vi "movestuff.vi"() -> ()   [LabVIEW 2017]
doc: "\"Discrete LED demo.vi\" -- Demonstrate a discrete LED connected to a digital output.\n\nInstructions:\n\n-- Click the 'enable blinker' button to toggle between blinking mode\nand static mode.\n-- In static mode, click the 'digital level' button to set the state of the\ndigital output.\n-- The 'digital output state' LED indicator shows the state of the\ndigital output (on = high, off = low)."
uses:
  <vilib>/myRIO/Instrument Drivers/Onboard IO/PWM/typedefs/PWM Reference.ctl
  <vilib>/myRIO/Common/Instrument Driver Framework/Utilities/typedefs/myRIO Generic Hardware Reference.ctl
  <vilib>/myRIO/Common/Instrument Driver Framework/Utilities/typedefs/Hardware Version Enum.ctl
  <vilib>/myRIO/Common/Instrument Driver Framework/Utilities/typedefs/myRIO v1.0 Reference.ctl
  <vilib>/myRIO/Common/Instrument Driver Framework/Utilities/typedefs/Generic FPGA Reference.ctl
  <vilib>/myRIO/Common/Instrument Driver Framework/myRIO v1.0/PWM/typedefs/PWM Channels Enum.ctl
  <vilib>/myRIO/Instrument Drivers/Onboard IO/PWM/typedefs/PWM Configuration.ctl
  <vilib>/userdefined/High Color/nirio_resource_hc.ctl
  <vilib>/myRIO/Instrument Drivers/Onboard IO/DIO/typedefs/DIO Reference.ctl
  <vilib>/myRIO/Common/Instrument Driver Framework/myRIO v1.0/DIO/typedefs/DIO Channels List.ctl
  <vilib>/myRIO/Common/Instrument Driver Framework/myRIO v1.0/DIO/typedefs/DIO Channels Enum.ctl
  <vilib>/myRIO/Common/Instrument Driver Framework/Utilities/vis/Is FPGA Ref Available.vi
  <vilib>/myRIO/Common/Instrument Driver Framework/myRIO v1.0/PWM/vis/myRIO v1.1 Open PWM.vi
  <vilib>/myRIO/Instrument Drivers/Onboard IO/PWM/vis/Set Duty Cycle and Frequency.vi
  <vilib>/myRIO/Common/Instrument Driver Framework/myRIO v1.0/DIO/vis/myRIO v1.1 Open DIO.vi
  <vilib>/myRIO/Instrument Drivers/Onboard IO/DIO/vis/Write.vi
  <vilib>/myRIO/Common/Instrument Driver Framework/Utilities/vis/Validate Channels.vi
  <vilib>/myRIO/Common/Instrument Driver Framework/myRIO v1.0/PWM/vis/myRIO v1.0 Reserve PWM.vi
  <vilib>/myRIO/Common/Instrument Driver Framework/myRIO v1.0/DIO/vis/myRIO v1.0 Reserve DIO.vi
  <vilib>/myRIO/Common/Instrument Driver Framework/myRIO v1.0/UART/vis/myRIO v1.0 Close UART.vi
  <vilib>/myRIO/Common/Instrument Driver Framework/myRIO v1.0/PWM/vis/myRIO v1.0 Build MUX Configuration PWM.vi
  <vilib>/myRIO/Common/Instrument Driver Framework/myRIO v1.0/Resource Manager/vis/myRIO v1.0 Reserve Channel List.vi
  <vilib>/myRIO/Common/Instrument Driver Framework/myRIO v1.0/DIO/vis/myRIO v1.0 Build MUX Configuration DIO.vi
  <vilib>/myRIO/Common/Instrument Driver Framework/myRIO v1.0/Resource Manager/vis/myRIO v1.0 Create Configuration List.vi
  <vilib>/myRIO/Common/Instrument Driver Framework/myRIO v1.0/Resource Manager/vis/myRIO v1.0 Reserve Channel.vi
  <vilib>/myRIO/Common/Instrument Driver Framework/myRIO v1.0/Resource Manager/vis/myRIO v1.0 Unreserve Channel.vi
  <vilib>/myRIO/Common/Instrument Driver Framework/myRIO v1.0/Resource Manager/vis/myRIO v1.0 Build Mutex Name.vi
  <vilib>/Utility/VariantDataType/GetNumericInfo.vi
  <vilib>/Utility/error.llb/Error Cluster From Error Code.vi
  <vilib>/myRIO/Common/Instrument Driver Framework/myRIO v1.0/myRIO v1.1 Open.vi
  <vilib>/myRIO/Common/Instrument Driver Framework/Utilities/vis/IO Manager.vi
  <vilib>/myRIO/Common/Instrument Driver Framework/Utilities/vis/Configuration Manager.vi
  <vilib>/myRIO/Common/Instrument Driver Framework/myRIO v1.0/Resource Manager/vis/myRIO v1.0 Configure IO.vi
  <vilib>/myRIO/Common/Instrument Driver Framework/myRIO v1.0/myRIO v1.0 Close.vi
  <vilib>/myRIO/Common/Instrument Driver Framework/myRIO v1.0/PWM/vis/myRIO v1.0 Write PWM.vi
  <vilib>/myRIO/Common/Instrument Driver Framework/myRIO v1.0/DIO/vis/myRIO v1.0 Write DIO.vi
  <vilib>/myRIO/Common/Instrument Driver Framework/Utilities/vis/FPGA Ref Manager.vi
  <vilib>/myRIO/Common/Instrument Driver Framework/myRIO v1.0/myRIO v1.0 Reset FPGA.vi
  <vilib>/myRIO/Common/Instrument Driver Framework/myRIO v1.0/IRQ/vis/myRIO v1.0 IRQ Info FGV.vi
  <vilib>/myRIO/Common/Instrument Driver Framework/myRIO v1.0/IRQ/vis/myRIO v1.0 Timer IRQ Info FGV.vi
  <vilib>/myRIO/Common/Instrument Driver Framework/myRIO v1.0/IRQ/vis/myRIO v1.0 ISR Agent.vi
  <vilib>/myRIO/Express VI/Onboard IO/PWM/PWM Express VI.xnode
  <vilib>/myRIO/Instrument Drivers/Onboard IO/PWM/vis/myRIO PWM Open.xnode
  <vilib>/myRIO/Express VI/Onboard Devices/LED/LED Express VI.xnode
  <vilib>/myRIO/Instrument Drivers/Onboard IO/DIO/vis/myRIO DIO Open.xnode
  <vilib>/myRIO/Express VI/Onboard IO/DO/DO Express VI.xnode
  <vilib>/myRIO/Instrument Drivers/Utilities/Utilities.lvlib
  <vilib>/myRIO/Instrument Drivers/Onboard IO/PWM/PWM.lvlib
  <vilib>/myRIO/Instrument Drivers/Onboard IO/DIO/DIO.lvlib
panel:
  in  "PWM 2":dbl(slide)=0.5 scale=0.0..1.0
  in  "PWM 1":dbl(slide)=0.5 scale=0.0..1.0
  in  "Stop Button":bool
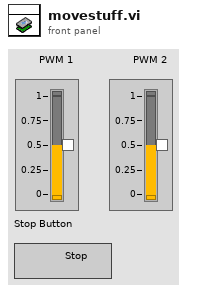
[diagram p1: front panel]
types:
  T1 = typedef "DIO.lvlib/DIO Reference.ctl" = cluster{"myRIO Reference":T2, "DIO Channels List":T6}
  T2 = typedef "myRIO Generic Hardware Reference.ctl" = cluster{"myRIO Model":T3, "myRIO Hardware Reference":T4}
  T3 = typedef "Hardware Version Enum.ctl" = enum16{"Unknown", "myRIO-1900", "myRIO-1950", "roboRIO", "NI ELVIS RIO CM"}
  T4 = typedef "myRIO v1.0 Reference.ctl" = cluster{"Generic FPGA Reference":T5, "Allow multiple opens":bool}
  T5 = typedef "Generic FPGA Reference.ctl" = refnum<k20>
  T6 = typedef "DIO Channels List.ctl" = T7[]
  T7 = typedef "DIO Channels Enum.ctl" = enum16{"Not Connected", "C/DIO0", "C/DIO1", "C/DIO2", "C/DIO3", "C/DIO4", "C/DIO5", "C/DIO6", "C/DIO7", "A/DIO0", "A/DIO1", "A/DIO2", "A/DIO3", "A/DIO4", "A/DIO5", "A/DIO6", "A/DIO7", "A/DIO8", "A/DIO9", "A/DIO10", "A/DIO11", "A/DIO12", "A/DIO13", "A/DIO14", "A/DIO15", "B/DIO0", "B/DIO1", "B/DIO2", "B/DIO3", "B/DIO4", "B/DIO5", "B/DIO6", "B/DIO7", "B/DIO8", "B/DIO9", "B/DIO10", "B/DIO11", "B/DIO12", "B/DIO13", "B/DIO14", "B/DIO15", "LED0", "LED1", "LED2", "LED3", "Button0", "DIO/DIO0", "DIO/DIO1", "DIO/DIO2", "DIO/DIO3", "DIO/DIO4", "DIO/DIO5", "DIO/DIO6", "DIO/DIO7", "DIO/DIO8", "DIO/DIO9", "SPI/CS0", "SPI/CS1", "SPI/CS2", "SPI/CS3", "LED RADIO (Green)", "LED RADIO (Red)", "LED COMM (Green)", "LED COMM (Red)", "LED MODE (Green)", "LED MODE (Red)"}
  T8 = typedef "nirio_resource_hc.ctl" = tag
  T9 = typedef "PWM.lvlib/PWM Reference.ctl" = cluster{"myRIO Reference":T2, "PWM Channels Enum":T10, "PWM Configuration":T11}
  T10 = typedef "PWM Channels Enum.ctl" = enum16{"Not Connected", "C/PWM0", "C/PWM1", "A/PWM0", "A/PWM1", "A/PWM2", "B/PWM0", "B/PWM1", "B/PWM2", "PWM/PWM0", "PWM/PWM1", "PWM/PWM2", "PWM/PWM3", "PWM/PWM4", "PWM/PWM5", "PWM/PWM6", "PWM/PWM7", "PWM/PWM8", "PWM/PWM9"}
  T11 = typedef "PWM.lvlib/PWM Configuration.ctl" = cluster{"Frequency":dbl, "Duty Cycle":dbl}
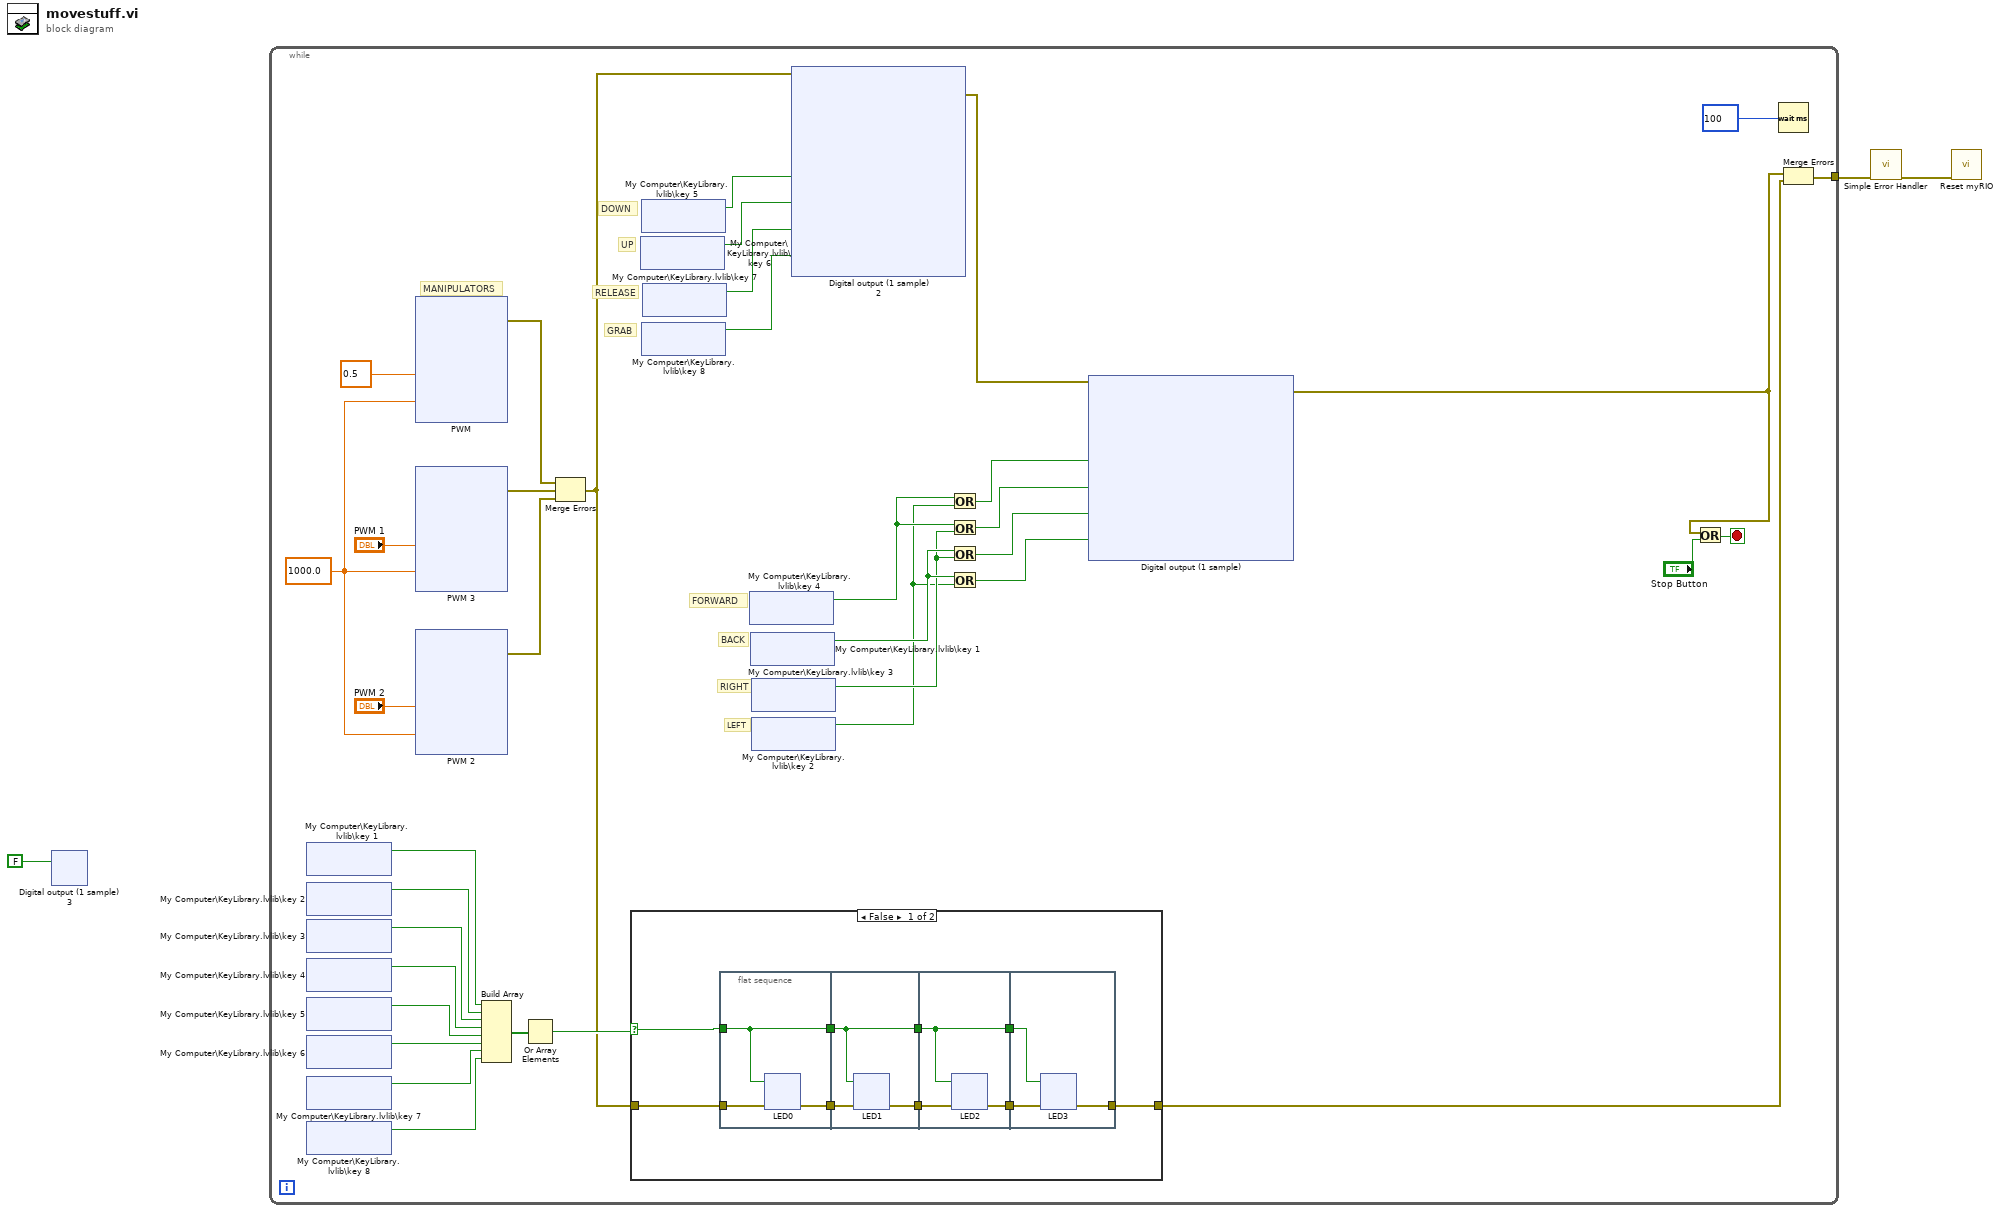
[diagram p0: block diagram]
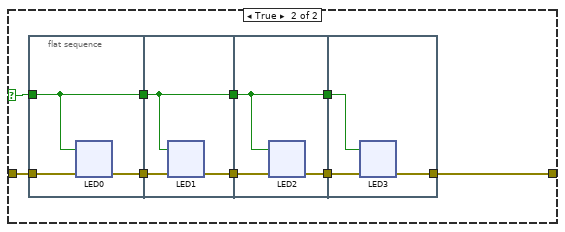
[diagram p2: hidden frame]
diagram:
  n1 = xnode "Digital output (1 sample) 3"("LED_pos (A/DIO2 (Pin 15))"=FALSE) -> ()  [unwired: 1 in, 1 out]
  n2 = while {
    tunnel: [w15] -> w2
    stop <- w39 stop-if-true
    w30 = 1000.0 ("Frequency [Hz]")
    # "RELEASE"
    # "GRAB"
    # "DOWN"
    # "UP"
    # "LEFT"
    # "RIGHT"
    # "BACK"
    # "FORWARD"
    # "MANIPULATORS"
    n3 = shared-variable "My Computer\\KeyLibrary.lvlib\\key 1"() -> (w25:bool)  [unwired: 1 in, 1 out]
    n4 = shared-variable "My Computer\\KeyLibrary.lvlib\\key 2"() -> (w24:bool)  [unwired: 1 in, 1 out]
    n5 = shared-variable "My Computer\\KeyLibrary.lvlib\\key 3"() -> (w23:bool)  [unwired: 1 in, 1 out]
    n6 = shared-variable "My Computer\\KeyLibrary.lvlib\\key 4"() -> (w22:bool)  [unwired: 1 in, 1 out]
    n7 = shared-variable "My Computer\\KeyLibrary.lvlib\\key 5"() -> (w21:bool)  [unwired: 1 in, 1 out]
    n8 = shared-variable "My Computer\\KeyLibrary.lvlib\\key 6"() -> (w20:bool)  [unwired: 1 in, 1 out]
    n9 = shared-variable "My Computer\\KeyLibrary.lvlib\\key 7"() -> (w19:bool)  [unwired: 1 in, 1 out]
    n10 = shared-variable "My Computer\\KeyLibrary.lvlib\\key 8"() -> (w18:bool)  [unwired: 1 in, 1 out]
    n11 = xnode "PWM"("Duty Cycle"=0.5, "Frequency [Hz]"=w30) -> ("error out"=w35:errorcluster)  [unwired: 1 in]
    n12 = xnode "PWM 3"("Duty Cycle"="PWM 1", "Frequency [Hz]"=w30) -> ("error out"=w38:errorcluster)  [unwired: 1 in]
    n13 = xnode "PWM 2"("Duty Cycle"="PWM 2", "Frequency [Hz]"=w30) -> ("error out"=w37:errorcluster)  [unwired: 1 in]
    n14 = Build Array(w25, w24, w23, w22, w21, w20, w19, w18) -> (w17:bool[])
    n15 = Or Array Elements(Boolean array=w17) -> (logical OR=w16:bool)
    n16 = Merge Errors(w35, w38, w37) -> (w13:errorcluster)
    n17 = case shown="False" w16 {
      selector: w16 -> [w41 w210]
      tunnel: [w42 w202] -> w14
      tunnel: w13 -> [w43 w203]
      frame False {
        n18 = flat-sequence {
          tunnel: w41 -> [w50]
          tunnel: [w50] -> w49
          tunnel: [w52] -> w48
          tunnel: w43 -> [w51]
          tunnel: [w90] -> w47
          tunnel: w49 -> [w90]
          tunnel: w48 -> [w89]
          tunnel: [w88] -> w46
          tunnel: [w128] -> w45
          tunnel: w47 -> [w128]
          tunnel: w46 -> [w127]
          tunnel: [w126] -> w44
          tunnel: w45 -> [w166]
          tunnel: w44 -> [w165]
          tunnel: [w164] -> w42
          frame #0 {
            n19 = xnode "LED0"("error in (no error)"=w51, "LED0"=w50) -> ("error out"=w52:errorcluster)
          }
          frame #1 {
            n20 = xnode "LED1"("error in (no error)"=w89, "LED1"=w90) -> ("error out"=w88:errorcluster)
          }
          frame #2 {
            n21 = xnode "LED2"("error in (no error)"=w127, "LED2"=w128) -> ("error out"=w126:errorcluster)
          }
          frame #3 {
            n22 = xnode "LED3"("error in (no error)"=w165, "LED3"=w166) -> ("error out"=w164:errorcluster)
          }
        }
      }
      frame True {
        n23 = flat-sequence {
          tunnel: w210 -> [w213]
          tunnel: [w213] -> w207
          tunnel: [w212] -> w206
          tunnel: w203 -> [w211]
          tunnel: [w251] -> w208
          tunnel: w207 -> [w251]
          tunnel: w206 -> [w250]
          tunnel: [w249] -> w205
          tunnel: [w289] -> w209
          tunnel: w208 -> [w289]
          tunnel: w205 -> [w288]
          tunnel: [w287] -> w204
          tunnel: w209 -> [w327]
          tunnel: w204 -> [w326]
          tunnel: [w325] -> w202
          frame #0 {
            n24 = xnode "LED0"("error in (no error)"=w211, "LED0"=w213) -> ("error out"=w212:errorcluster)
          }
          frame #1 {
            n25 = xnode "LED1"("error in (no error)"=w250, "LED1"=w251) -> ("error out"=w249:errorcluster)
          }
          frame #2 {
            n26 = xnode "LED2"("error in (no error)"=w288, "LED2"=w289) -> ("error out"=w287:errorcluster)
          }
          frame #3 {
            n27 = xnode "LED3"("error in (no error)"=w326, "LED3"=w327) -> ("error out"=w325:errorcluster)
          }
        }
      }
    }
    n28 = shared-variable "My Computer\\KeyLibrary.lvlib\\key 6"() -> (w6:bool)  [unwired: 1 in, 1 out]
    n29 = shared-variable "My Computer\\KeyLibrary.lvlib\\key 5"() -> (w7:bool)  [unwired: 1 in, 1 out]
    n30 = shared-variable "My Computer\\KeyLibrary.lvlib\\key 8"() -> (w4:bool)  [unwired: 1 in, 1 out]
    n31 = shared-variable "My Computer\\KeyLibrary.lvlib\\key 7"() -> (w5:bool)  [unwired: 1 in, 1 out]
    n32 = shared-variable "My Computer\\KeyLibrary.lvlib\\key 4"() -> (w29:bool)  [unwired: 1 in, 1 out]
    n33 = shared-variable "My Computer\\KeyLibrary.lvlib\\key 1"() -> (w28:bool)  [unwired: 1 in, 1 out]
    n34 = shared-variable "My Computer\\KeyLibrary.lvlib\\key 3"() -> (w9:bool)  [unwired: 1 in, 1 out]
    n35 = shared-variable "My Computer\\KeyLibrary.lvlib\\key 2"() -> (w8:bool)  [unwired: 1 in, 1 out]
    n36 = xnode "Digital output (1 sample) 2"("M+ (B/DIO5 (Pin 21))"=w7, "M- (B/DIO6 (Pin 23))"=w6, "G+ (B/DIO7 (Pin 25))"=w5, "G- (B/DIO13 (Pin 26))"=w4, "error in (no error)"=w13) -> ("error out"=w33:errorcluster)
    n37 = Or(x=w29, y=w8) -> (x .or. y?=w27:bool)
    n38 = Or(x=w29, y=w9) -> (x .or. y?=w10:bool)
    n39 = Or(x=w28, y=w9) -> (x .or. y?=w11:bool)
    n40 = Or(x=w28, y=w8) -> (x .or. y?=w26:bool)
    n41 = xnode "Digital output (1 sample)"("Left+ (A/DIO5 (Pin 21))"=w27, "Right+ (A/DIO7 (Pin 25))"=w10, "Left- (A/DIO6 (Pin 23))"=w11, "Right- (A/DIO13 (Pin 26))"=w26, "error in (no error)"=w33) -> ("error out"=w12:errorcluster)
    n42 = Or(x=w12, y="Stop Button") -> (x .or. y?=w39:bool)
    n43 = Wait (ms)(milliseconds to wait=u32 100 ("millisecond timer value")) -> ()  [unwired: 1 out]
    n44 = Merge Errors(w12, w14) -> (w15:errorcluster)
  }
  n45 = call <vilib>:"Simple Error Handler.vi"("error in (no error)"=w2) -> ("error out"=w3:errorcluster)  [unwired: 4 in, 4 out]
  n46 = call <vilib>:"Reset myRIO.vi"("error in (no error)"=w3) -> ()  [unwired: 10 in, 1 out]
